vi "Ordering System.vi"() -> ()   [LabVIEW 2024]
panel:
  in  "Dashboard":enum32{"Order Placement", "Order Confirmation"}(tab)
  out "Total dishes selected":string
  out "Menu":cluster{"Price":dbl, "Dish Name":string}[](array[cluster])
  in  "Quantity of Each Item":cluster{"Quantity":dbl}[](array[cluster])
  in  "Confirm Order":bool
  in  "Stop":bool
  out "Grand Total Amount":string
  out "Total Items Orderd":string
  in  "Place Order !":bool
  in  "Make Changes":bool
  out "Final Order":T1(array[cluster])
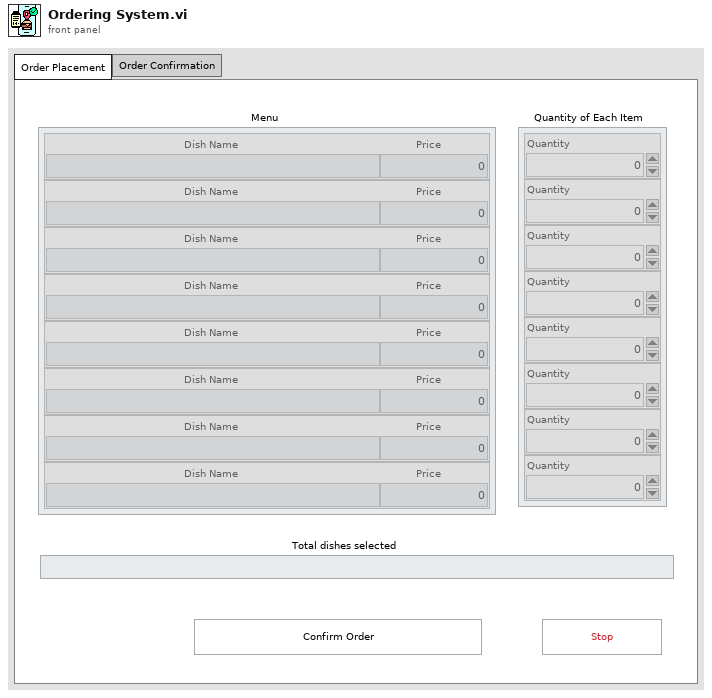
[diagram p1: front panel]
types:
  T1 = cluster{"Dish Name":string, "Price":dbl, "Quantity":dbl, "Total Cost":dbl}[]
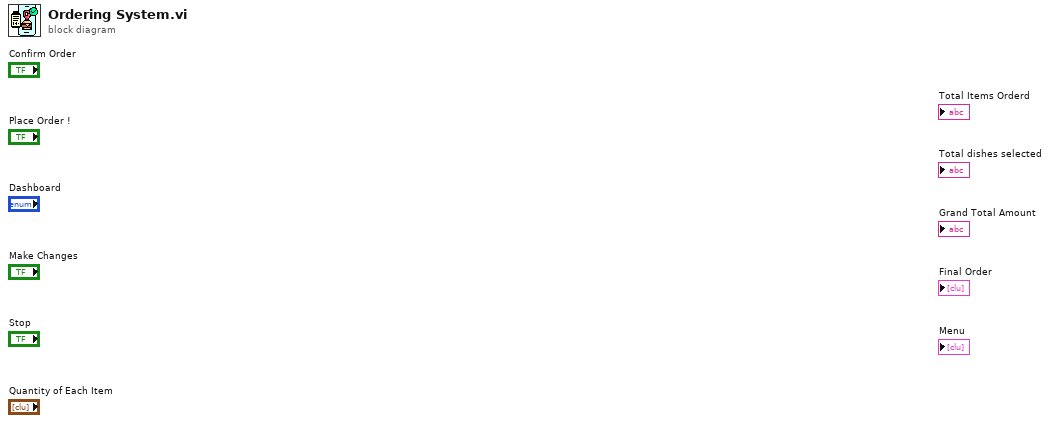
[diagram p0: block diagram]
diagram:
